vi "Get Server.vi"(8 "error in (no error)":errorcluster, 11 "Handler in":refnum<class "Handler.lvclass">) -> (0 "error out":errorcluster, 3 "Base Server":refnum<class "Server.lvclass">)   [LabVIEW 2024, in "Ramses Framework.lvlib" / "Handler.lvclass"]
uses:
  Handler.lvclass
  Base Server/Server.lvclass
  Handler.lvclass/Handler.ctl
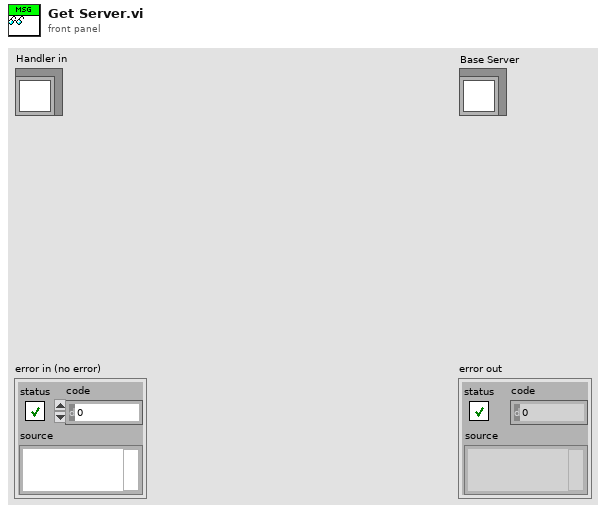
[diagram p1: front panel]
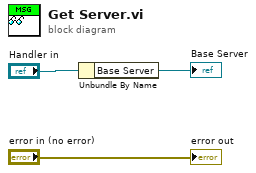
[diagram p0: block diagram]
diagram:
  n1 = Unbundle By Name("Handler in") -> ("Base Server"=→"Base Server":refnum<class "Server.lvclass">)
  "error out" <- "error in (no error)"
